vi "HFRR ADV v026 new software.vi"() -> ()   [LabVIEW 2025] (continued)
                n2409 = And(x=w2959, y=w2958) -> (x .and. y?=w2960:bool)
                n2410 = Not(x="Engage") -> (.not. x?=w2949:bool)
                n2411 = case shown="False" w2943 {
                  tunnel: [0.0 w2989] -> w2945
                  frame False {
                    (unwired) TRUE ("Visible")
                    n2412 = local read "Auto Start Test"() -> (w2970:bool)
                    n2413 = local write "Start Time"(TRUE ("Start Time")) -> ()
                    n2414 = property on="Stroke 2" class="DigNum (strict)"("Visible"=FALSE) -> ()  [unwired: 2 in, 2 out]
                    n2415 = case shown="False" w2970 {
                      frame False {
                        n2416 = property on="Heater Button" class="Bool (strict)"("DisabledEnum"=T18."Enabled" ("Disabled")) -> ()  [unwired: 2 in, 2 out]
                        n2417 = property on="Humidity" class="Bool (strict)"("DisabledEnum"=T18."Enabled" ("Disabled")) -> ()  [unwired: 2 in, 2 out]
                      }
                      frame True {
                      }
                    }
                    n2418 = case shown="False" "TestCompFlg" {
                      frame False {
                        n2419 = local read "StartFlg"() -> (w2978:bool)
                        n2420 = case shown="True" w2978 {
                          frame False {
                          }
                          frame True {
                            n2421 = stacked-sequence {
                              frame #0 {
                                n2422 = local read "EVENT LOG"() -> (w2982:string)
                                n2423 = call "Event Log.vi"("Content"="Test was interrupted", "EVENT LOG"=w2982) -> ("EVENT LOG"=w2983:string)  [unwired: 8 in, 1 out]
                                n2424 = local write "EVENT LOG"(w2983) -> ()
                                n2425 = property on="RUN" class="Bool (strict)"("Visible"=TRUE) -> ()  [unwired: 2 in, 2 out]
                                n2426 = property on="Auto Start Test" class="Bool (strict)"("Visible"=TRUE) -> ()  [unwired: 2 in, 2 out]
                              }
                              frame #1 {
                                w2985 = FALSE ("StartFlg")
                                n2427 = property on="Heater Button" class="Bool (strict)"("Val(Sgnl)"=FALSE ("Value (Signaling)")) -> ()  [unwired: 2 in, 2 out]
                                n2428 = local write "Heater Button"(w2985) -> ()
                                n2429 = local write "StartFlg"(w2985) -> ()
                                n2430 = local write "Humidity"(w2985) -> ()
                              }
                              frame #2 {
                                n2431 = local write "Due Write"("VC;0" ("Command")) -> ()
                              }
                              frame #3 {
                                n2432 = Wait (ms)(milliseconds to wait=u32 1500) -> ()  [unwired: 1 out]
                              }
                              frame #4 {
                                n2433 = local write "Due Write"("HE;0" ("Command")) -> ()
                              }
                            }
                          }
                        }
                      }
                      frame True {
                      }
                    }
                    n2434 = local write "String 14"("Test will autostart once parameters reach the set value." ("String 14")) -> ()
                  }
                  frame True {
                    (unwired) FALSE ("Visible")
                    n2435 = property on="Stroke 2" class="DigNum (strict)"("Visible"=TRUE) -> ()  [unwired: 2 in, 2 out]
                    n2436 = property on="STOP 2" class="Bool (strict)"("Disabled"=u8 2) -> ()  [unwired: 2 in, 2 out]
                    n2437 = local write "String 14"(" Running....." ("String 14")) -> ()
                    n2438 = property on="Heater Button" class="Bool (strict)"("DisabledEnum"=T18."Disabled and Grayed Out" ("Disabled")) -> ()  [unwired: 2 in, 2 out]
                    n2439 = property on="Humidity" class="Bool (strict)"("DisabledEnum"=T18."Disabled and Grayed Out" ("Disabled")) -> ()  [unwired: 2 in, 2 out]
                    n2440 = case shown="True" "Start Time" {
                      selector: "Start Time" -> [_ w3008]
                      frame False {
                      }
                      frame True {
                        n2441 = Not(x=w3008) -> (.not. x?=w3007:bool)
                        n2442 = local write "Start Time"(w3007) -> ()
                        n2443 = local read "EVENT LOG"() -> (w3009:string)
                        n2444 = call "Event Log.vi"("Content"="Test in progress", "EVENT LOG"=w3009) -> ("EVENT LOG"=w3011:string)  [unwired: 8 in, 1 out]
                        n2445 = local write "EVENT LOG"(w3011) -> ()
                      }
                    }
                    n2446 = disable-structure shown="Enabled" {
                      disable-tunnel: [w3000 w3006] -> w2989
                      frame Disabled {
                        n2447 = local read "Set Hz"() -> (w3003:dbl)
                        n2448 = call <vilib>:"Uniform White Noise Waveform.vi"() -> ("signal out"=w3002:waveform(dbl))  [unwired: 10 in, 1 out]
                        n2449 = Random Number (0-1)() -> (number: 0 to 1=w2999:dbl)
                        n2450 = Add(x=w3003, y=w3002) -> (x+y=w3001:waveform(dbl))
                        n2451 = Multiply(x=ext 0.01 ("y"), y=w2999) -> (x*y=w2997:ext)
                        n2452 = Multiply(x=w3001, y=w2997) -> (x*y=w3000:waveform(ext))
                      }
                      frame Enabled {
                        n2453 = call-poly <vilib>:"Random Number (Range).vi"("lower bound (0)"=49.89, "upper bound (100)"=50.8) -> ("number"=w3006:dbl)  [unwired: 9 in]
                      }
                    }
                    "StartFlg" <- TRUE ("StartFlg")
                  }
                }
                n2454 = case shown="True" w2960 {
                  frame False {
                  }
                  frame True {
                    n2455 = local write "clk"(10.0 ("clk")) -> ()
                    n2456 = Get Date/Time In Seconds() -> (seconds since 1Jan1904=w3014:timestamp)
                    n2457 = To Double Precision Float(number=w3014) -> (double precision float=w3012:dbl)
                    n2458 = local write "acq timer"(w3012) -> ()
                    n2459 = local write "act save time"(w3012) -> ()
                  }
                }
                n2460 = call "Elapsed Time"("Time Target (s)"="Countdown", "Reset"=w2949) -> ("Elapsed Time (s)"=w2954:dbl, "Time has Elapsed"=w2952:bool)  [unwired: 10 in, 6 out]
                "Countdown 2" <- w2954
                n2461 = Subtract(x=w2954, y=2.0) -> (x-y=w2957:dbl)
                n2462 = Less?(x=w2957, y="Countdown") -> (x < y?=w2955:bool)
                n2463 = And(x=w2955, y=w2952) -> (x .and. y?=w2951:bool)
                n2464 = case shown="True" w2951 {
                  frame False {
                  }
                  frame True {
                    (unwired) dbl[] [] ("History Data")
                    n2465 = local write "Engage"(FALSE ("Engage")) -> ()
                    n2466 = local write "RUN"(TRUE ("RUN")) -> ()
                    n2467 = local read "Humidity ( %RH )"() -> (→"Rh Before":dbl)
                  }
                }
                n2468 = local read "Test \nStatus"() -> (w2947:bool)
                n2469 = Select(t=w2945, s=w2947, f=0.0) -> (s? t:f=w2946:dbl)
                n2470 = local write "Frequency ( Hz )"(w2946) -> ()
              }
              frame #1 {
                w3037 = 1000000.0 ("x")
                # "HC;1/0\nST;VALUE"
                # "Elapsed time\ncof\nstroke\nAir temp\nTemp\nHumidity"
                # "acq timer\n\nact save time"
                # "convert to microseconds"
                n2471 = local read "COUNT"() -> (w3020:i32)
                n2472 = local read "Rate"() -> (w3033:dbl)
                n2473 = Divide(x=w3037, y=w3033) -> (x/y=w3038:dbl)
                n2474 = Greater Or Equal?(x=w3020, y=250) -> (x >= y?=w3019:bool)
                n2475 = Get Date/Time In Seconds() -> (seconds since 1Jan1904=w3040:timestamp)
                n2476 = case shown="True" w3019 {
                  frame False {
                    n2477 = local read "COUNT"() -> (w3041:i32)
                    n2478 = Increment(x=w3041) -> (x+1=w3042:i32)
                    n2479 = local write "COUNT"(w3042) -> ()
                  }
                  frame True {
                    n2480 = local write "COUNT"(0 ("COUNT")) -> ()
                  }
                }
                n2481 = local read "Samplingtime 2"() -> (w3018:dbl)
                n2482 = local read "act save time"() -> (w3035:dbl)
                n2483 = Divide(x=w3038, y=w3037) -> (x/y=w3036:dbl)
                n2484 = To Double Precision Float(number=w3040) -> (double precision float=w3029:dbl)
                n2485 = Add(x=w3035, y=w3018) -> (x+y=w3034:dbl)
                n2486 = local read "acq timer"() -> (w3039:dbl)
                n2487 = local read "COUNT"() -> (w3022:i32)
                n2488 = Greater Or Equal?(x=w3029, y=w3034) -> (x >= y?=w3017:bool)
                n2489 = Multiply(x=w3036, y=w3022) -> (x*y=w3028:dbl)
                n2490 = Subtract(x=w3029, y=w3039) -> (x-y=w3031:dbl)
                n2491 = local read "Save"() -> (w3032:bool)
                n2492 = Add(x=w3031, y=w3028) -> (x+y=w3015:dbl)
                "Elapsed time 3" <- w3015
                n2493 = And(x=w3017, y=w3032) -> (x .and. y?=w3030:bool)
                n2494 = Divide(x=w3015, y=60.0) -> (x/y=w3026:dbl)
                n2495 = local read "Test \nStatus"() -> (w3016:bool)
                n2496 = local read "clk"() -> (w3023:dbl)
                n2497 = Equal?(x=w3023, y=10.0) -> (x = y?=w3025:bool)
                n2498 = case shown="True" w3030 {
                  tunnel: w3029 -> [_ w3153]
                  tunnel: [FALSE ("Boolean 2") TRUE ("Boolean 2")] -> _
                  frame False {
                  }
                  frame True {
                    w3107 = ";" ("Substring")
                    # "Pid out/\nFreq response value"
                    n2499 = local write "act save time"(w3153) -> ()
                    n2500 = local read "FILE"() -> (w3101:string)
                    n2501 = call "file check.vi"("file name in"=w3101) -> ("error out"=w3104:errorcluster, "file name out"=w3099:string)  [unwired: 9 in]
                    n2502 = local read "LVDT STROKE"() -> (w3096:dbl)
                    n2503 = local read "Add up Stroke"() -> (w3094:dbl)
                    n2504 = call "FILE PATH CREATION.vi"("error in"=w3104, "FILE NAME :"=w3099) -> ("FILE OUT"=w3102:path)  [unwired: 8 in, 1 out]
                    n2505 = Concatenate Strings(w3099, ".dgf" ("Substring")) -> (w3103:string)
                    n2506 = Subtract(x=w3096, y=w3094) -> (x-y=w3095:dbl)
                    n2507 = Absolute Value(x=w3095) -> (abs(x)=w3093:dbl)
                    n2508 = local read "FF 2"() -> (→"Frictional Force ( N )" →"Frictional Force ( N )":dbl)
                    n2509 = Build Path(base path=w3102, name or relative path=w3103) -> (appended path=w3098:path)
                    n2510 = local read "COF 2"() -> (w3112:dbl)
                    "Coefficient of Friction" <- w3112
                    "COF 4" <- w3112
                    "Coefficient of Friction" <- w3112
                    n2511 = local read "TEMP"() -> (w3115:dbl)
                    "Temperature ( Deg C )" <- w3115
                    n2512 = local read "Humidity ( %RH )"() -> (w3114:dbl)
                    "Humidity ( %RH )" <- w3114
                    "Humidity ( %RH )" <- w3114
                    n2513 = local read "Frequency ( Hz )"() -> (w3121:dbl)
                    n2514 = call <vilib>:"Mean PtByPt.vi"("x"=w3093, "sample length"="STROKE FILTER") -> ("mean"=w3092:dbl)  [unwired: 2 in, 1 out]
                    n2515 = local read "Elapsed time"() -> (w3146:dbl)
                    n2516 = local read "AIR TEMP"() -> (w3119:dbl)
                    n2517 = local read "PID-out"() -> (w3124:dbl)
                    n2518 = local write "Temperature ( Deg C )"(w3115) -> ()
                    n2519 = Number To Fractional String(number=w3092, width (-)=i16 9 ("precision (6)"), precision (6)=i16 6) -> (F-format string=w3139:string)  [unwired: 1 in]
                    n2520 = Number To Fractional String(number=w3119, width (-)=i16 9 ("precision (6)"), precision (6)=i16 3) -> (F-format string=w3138:string)  [unwired: 1 in]
                    n2521 = Number To Fractional String(number=w3115, width (-)=i16 9 ("precision (6)"), precision (6)=i16 3) -> (F-format string=w3135:string)  [unwired: 1 in]
                    n2522 = Number To Fractional String(number=w3114, width (-)=i16 9 ("precision (6)"), precision (6)=i16 3) -> (F-format string=w3132:string)  [unwired: 1 in]
                    n2523 = Number To Fractional String(number=0.0, width (-)=i16 9 ("precision (6)"), precision (6)=i16 3) -> (F-format string=w3129:string)  [unwired: 1 in]
                    n2524 = Number To Fractional String(number=w3124, width (-)=i16 9 ("precision (6)"), precision (6)=i16 3) -> (F-format string=w3125:string)  [unwired: 1 in]
                    n2525 = Number To Fractional String(number=w3121, width (-)=i16 9 ("precision (6)"), precision (6)=i16 3) -> (F-format string=w3120:string)  [unwired: 1 in]
                    n2526 = Number To Fractional String(number=w3112, width (-)=i16 9 ("precision (6)"), precision (6)=i16 6) -> (F-format string=w3147:string)  [unwired: 1 in]
                    n2527 = Number To Fractional String(number=w3146, width (-)=i16 14 ("precision (6)"), precision (6)=i16 3) -> (F-format string=w3148:string)  [unwired: 1 in]
                    n2528 = Bundle("y"=1.02, "mean"=w3092, "y"=0.98) -> (w3113:cluster{"y":dbl, "mean":dbl, "y":dbl})  [unwired: 1 in]
                    n2529 = Number To Fractional String(number="Ambient Humidity :", width (-)=i16 9 ("precision (6)"), precision (6)=i16 6) -> (F-format string=w3105:string)  [unwired: 1 in]
                    n2530 = local read "RUN"() -> (w3111:bool)
                    n2531 = case shown="True" w3111 {
                      tunnel: w3113 -> [_ w3158]
                      tunnel: w3092 -> [_ w3157]
                      tunnel: w3092 -> [_ w3155]
                      tunnel: w3092 -> [_ w3156]
                      frame False {
                      }
                      frame True {
                        "Stroke ( mm )" <- w3158
                        "Stroke ( mm )" <- w3158
                        "Stroke 4" <- w3157
                        "Stroke 3" <- w3155
                        "Stroke 2" <- w3156
                        "measured_stroke" <- w3155
                      }
                    }
                    n2532 = Concatenate Strings(w3148, w3107, w3147, w3107, w3139, w3107, w3138, w3107, w3135, w3107, w3132, w3107, w3129, w3107, w3125, w3107, w3120, w3107, w3105, "\r") -> (w3145:string)
                    n2533 = call <vilib>:"Write Characters To File.vi"("append to file? (new file:F)"=TRUE, "character string"=w3145, "file path (dialog if empty)"=w3098) -> ()  [unwired: 2 in, 1 out]
                    "refresh flag" <- TRUE ("refresh flag")
                  }
                }
                n2534 = case shown="True" w3016 {
                  tunnel: w3026 -> [_ w3052]
                  tunnel: w3031 -> [_ w3062]
                  tunnel: [0.0 w3058] -> _
                  tunnel: w3025 -> [_ w3057]
                  tunnel: [0.0 w3056] -> _
                  tunnel: w3015 -> [_ w3056]
                  tunnel: w3029 -> [w3045 _]
                  frame False {
                    n2535 = local write "acq timer"(w3045) -> ()
                    n2536 = local write "Test Duration Status"(0.0 ("Test Duration Status")) -> ()
                  }
                  frame True {
                    n2537 = local read "Set Hz"() -> (w3059:dbl)
                    n2538 = local write "Elapsed time"(w3052) -> ()
                    n2539 = local read "test time"() -> (w3051:dbl)
                    n2540 = Multiply(x=w3062, y=w3059) -> (x*y=w3061:dbl)
                    n2541 = case shown="False" w3057 {
                      tunnel: w3061 -> [w3063 _]
                      tunnel: [w3063 1.0] -> w3058
                      frame False {
                        n2542 = local write "Cycles elapsed"(w3063) -> ()
                      }
                      frame True {
                      }
                    }
                    n2543 = Greater?(x=w3052, y=w3051) -> (0:w3060:bool)
                    n2544 = Subtract(x=w3051, y=w3052) -> (x-y=w3050:dbl)
                    n2545 = Multiply(x=w3050, y=60.0) -> (x*y=w3049:dbl)
                    n2546 = local write "Time Remaining"(w3049) -> ()
                    n2547 = local write "Remaining Time"(w3049) -> ()
                    n2548 = case shown="True" w3060 {
                      frame False {
                      }
                      frame True {
                        n2549 = stacked-sequence {
                          frame #0 {
                            w3068 = T18."Enabled" ("Disabled")
                            w3067 = FALSE ("TEST FILE NAM,E SAVED")
                            w3069 = "" ("FILE")
                            w3070 = TRUE ("Visible")
                            n2550 = local write "Humidity"(FALSE ("Humidity")) -> ()
                            n2551 = local write "RUN"(FALSE ("OK Button 2")) -> ()
                            n2552 = local write "Heater Button"(FALSE ("Heater Button")) -> ()
                            n2553 = local write "Auto Start Test"(FALSE ("Auto Start Test")) -> ()
                            n2554 = local write "TestCompFlg"(TRUE ("StpFlg")) -> ()
                            n2555 = local read "Humidity ( %RH )"() -> (→"Rh After":dbl)
                            n2556 = property on="STOP 2" class="Bool (strict)"("Disabled"=u8 0) -> ()  [unwired: 2 in, 2 out]
                            n2557 = local read "EVENT LOG"() -> (w3075:string)
                            n2558 = call "Event Log.vi"("Content"="Test Completed", "EVENT LOG"=w3075) -> ("EVENT LOG"=w3074:string)  [unwired: 8 in, 1 out]
                            n2559 = property on="RUN" class="Bool (strict)"("Visible"=w3070) -> ()  [unwired: 2 in, 2 out]
                            n2560 = property on="Auto Start Test" class="Bool (strict)"("Visible"=w3070) -> ()  [unwired: 2 in, 2 out]
                            n2561 = local write "Batch Ref Num :"(w3069) -> ()
                            n2562 = local write "FILE"(w3069) -> ()
                            n2563 = local write "EVENT LOG"(w3074) -> ()
                            n2564 = local write "TEST FILE NAM,E SAVED"(w3067) -> ()
                            n2565 = local write "Fuel Discription :"(w3069) -> ()
                            n2566 = local write "START TEMP"(w3067) -> ()
                            n2567 = local write "Remarks :"(w3069) -> ()
                            n2568 = local write "Main Dashboard Buttons"(T1."Imaging" ("Main Dashboard Buttons")) -> ()
                            n2569 = local write "Main Tab"(T2."Adv Scar" ("Main Tab")) -> ()
                            n2570 = property on="FRICVALZ 2" class="Bool (strict)"("DisabledEnum"=w3068) -> ()  [unwired: 2 in, 2 out]
                            n2571 = property on="FRICVALZ 3" class="Bool (strict)"("DisabledEnum"=w3068) -> ()  [unwired: 2 in, 2 out]
                            n2572 = property on="FRICVALZ 4" class="Bool (strict)"("DisabledEnum"=w3068) -> ()  [unwired: 2 in, 2 out]
                          }
                          frame #1 {
                            n2573 = Wait (ms)(milliseconds to wait=u32 1500) -> ()  [unwired: 1 out]
                          }
                          frame #2 {
                            n2574 = local write "Due Write"("VC;0") -> ()
                          }
                          frame #3 {
                            n2575 = Wait (ms)(milliseconds to wait=u32 1500) -> ()  [unwired: 1 out]
                          }
                          frame #4 {
                            n2576 = local write "Due Write"("VC;0") -> ()
                          }
                          frame #5 {
                            n2577 = Wait (ms)(milliseconds to wait=u32 1500) -> ()  [unwired: 1 out]
                          }
                          frame #6 {
                            n2578 = local write "Due Write"("ST;0") -> ()
                          }
                          frame #7 {
                            n2579 = local write "measured_stroke"(0.0 ("measured_stroke")) -> ()
                            n2580 = Wait (ms)(milliseconds to wait=u32 1500) -> ()  [unwired: 1 out]
                          }
                          frame #8 {
                            n2581 = local write "Due Write"("HE;0") -> ()
                          }
                        }
                      }
                    }
                    n2582 = Divide(x=w3052, y=w3051) -> (x/y=w3055:dbl)
                    n2583 = Multiply(x=w3055, y=100.0) -> (x*y=w3053:dbl)
                    n2584 = local write "Test Duration Status"(w3053) -> ()
                  }
                }
              }
              frame #2 {
                n2585 = case shown="True" "Heater Button" {
                  tunnel: [0.0 ("output") w3181] -> w3159
                  frame False {
                    w3162 = TRUE ("tmpchk")
                    n2586 = local read "TEMP"() -> (w3163:dbl)
                    n2587 = local write "Temp ini"(w3163) -> ()
                    n2588 = local write "Reset 4"(w3162) -> ()
                    n2589 = local write "tmpchk"(w3162) -> ()
                    n2590 = local write "reinit"(TRUE ("reinit")) -> ()
                    n2591 = local write "manual temp log"(TRUE ("manual temp log")) -> ()
                  }
                  frame True {
                    # "Logic to turn off\nthe heater when \ntemp is not rising.\nTime - 60 sec\nDelta t- 5°c"
                    n2592 = local read "Temp ini"() -> (w3170:dbl)
                    n2593 = local read "Auto Start Test"() -> (w3166:bool)
                    n2594 = Less?(x=w3170, y=53.0) -> (x < y?=w3168:bool)
                    n2595 = case shown="False" w3166 {
                      frame False {
                        n2596 = local read "Set Temp"() -> (w3190:dbl)
                        n2597 = local read "TEMP"() -> (w3189:dbl)
                        n2598 = Subtract(x=w3190, y=w3189) -> (x-y=w3188:dbl)
                        n2599 = Absolute Value(x=w3188) -> (abs(x)=w3187:dbl)
                        n2600 = Less?(x=w3187, y=0.5) -> (x < y?=w3185:bool)
                        n2601 = case shown="True" w3185 {
                          tunnel: "manual temp log" -> [_ w3191]
                          frame False {
                          }
                          frame True {
                            n2602 = case shown="True" w3191 {
                              selector: w3191 -> [_ w3192]
                              frame False {
                              }
                              frame True {
                                # "#Event log"
                                n2603 = Not(x=w3192) -> (.not. x?=w3193:bool)
                                n2604 = local write "manual temp log"(w3193) -> ()
                                n2605 = local read "EVENT LOG"() -> (w3196:string)
                                n2606 = call "Event Log.vi"("Content"="Target Temperature reached", "EVENT LOG"=w3196) -> ("EVENT LOG"=w3195:string)  [unwired: 8 in, 1 out]
                                n2607 = local write "EVENT LOG"(w3195) -> ()
                              }
                            }
                          }
                        }
                      }
                      frame True {
                        n2608 = local write "manual temp log"(TRUE ("manual temp log")) -> ()
                      }
                    }
                    n2609 = And(x="tmpchk", y=w3168) -> (x .and. y?=w3171:bool)
                    n2610 = case shown="True" w3171 {
                      frame False {
                      }
                      frame True {
                        n2611 = call "Elapsed Time8"("Time Target (s)"=300.0, "Reset"="Reset 4") -> ("Time has Elapsed"=w3198:bool)  [unwired: 10 in, 7 out]
                        n2612 = flat-sequence {
                          tunnel: w3198 -> [_]
                          frame #0 {
                            n2613 = local write "Reset 4"(FALSE ("Reset 4")) -> ()
                          }
                        }
                        n2614 = case shown="True" w3198 {
                          frame False {
                          }
                          frame True {
                            n2615 = local read "Temp ini"() -> (w3205:dbl)
                            n2616 = Add(x=w3205, y=5.0) -> (x+y=w3203:dbl)
                            n2617 = local read "TEMP"() -> (w3206:dbl)
                            n2618 = Greater?(x=w3206, y=w3203) -> (0:w3204:bool)
                            n2619 = case shown="False" w3204 {
                              frame False {
                                n2620 = local write "Heater Button"(FALSE ("Heater Button")) -> ()
                              }
                              frame True {
                                n2621 = local write "tmpchk"(FALSE ("tmpchk")) -> ()
                              }
                            }
                          }
                        }
                      }
                    }
                    n2622 = local read "Set Temp"() -> (w3179:dbl)
                    n2623 = local read "TEMP"() -> (w3173:dbl)
                    n2624 = call-poly <vilib>:"PID.vi"("reinitialize? (F)"="reinit", "dt (s)"=-1.0, "process variable"=w3173, "setpoint"=w3179) -> ("output"=w3176:dbl)  [unwired: 6 in, 1 out]
                    n2625 = Subtract(x=w3179, y=w3173) -> (x-y=w3180:dbl)
                    n2626 = Add(x=w3179, y=0.5) -> (x+y=w3177:dbl)
                    n2627 = Greater Or Equal?(x=w3173, y=w3177) -> ()  [unwired: 1 out]
                    n2628 = Select(t=0.0, s=FALSE, f=w3176) -> (s? t:f=w3175:dbl)
                    "PID output" <- w3175
                    n2629 = flat-sequence {
                      tunnel: w3175 -> [w3209]
                      tunnel: [w3209] -> w3181
                      frame #0 {
                        n2630 = local write "reinit"(FALSE ("reinit")) -> ()
                      }
                    }
                    n2631 = Bundle(w3180, "output"=w3175, "TEMP"=w3173) -> ()  [unwired: 1 in, 1 out]
                  }
                }
                "PID-out" <- w3159
              }
              frame #3 {
                n2632 = local read "TEMP"() -> (w3211:dbl)
                n2633 = Greater Or Equal?(x=w3211, y="Set Temp 2") -> (x >= y?=w3216:bool)
                n2634 = case shown="True" w3216 {
                  tunnel: [FALSE TRUE] -> w3214
                  frame False {
                  }
                  frame True {
                  }
                }
                "Status 13" <- w3214
                n2635 = And(x=w3214, y="trip1 8") -> (x .and. y?=w3213:bool)
                n2636 = case shown="True" w3213 {
                  frame False {
                    n2637 = local write "Heater Trip Temp"(TRUE ("Heater Trip Temp")) -> ()
                  }
                  frame True {
                    w3219 = FALSE ("OK Button 2")
                    n2638 = case shown="True" "Heater Trip Temp" {
                      selector: "Heater Trip Temp" -> [_ w3221]
                      frame False {
                      }
                      frame True {
                        n2639 = Not(x=w3221) -> (.not. x?=w3220:bool)
                        n2640 = local read "EVENT LOG"() -> (w3224:string)
                        n2641 = local write "Heater Trip Temp"(w3220) -> ()
                        n2642 = call "Event Log.vi"("Content"="Heater Trip", "EVENT LOG"=w3224) -> ("EVENT LOG"=w3223:string)  [unwired: 8 in, 1 out]
                        n2643 = local write "EVENT LOG"(w3223) -> ()
                      }
                    }
                    n2644 = local write "RUN"(w3219) -> ()
                    n2645 = property on="Auto Start Test" class="Bool (strict)"("Value"=w3219) -> ()  [unwired: 2 in, 2 out]
                    n2646 = local write "Heater Button"(w3219) -> ()
                  }
                }
              }
            }
            n2647 = case shown="False" w2940 {
              frame False {
                n2648 = disable-structure shown="Disabled" {
                  frame Disabled {
                    n2649 = stacked-sequence {
                      frame #0 {
                        n2650 = local write "RUN"(FALSE ("OK Button 2")) -> ()
                      }
                      frame #1 {
                      }
                    }
                  }
                  frame Enabled {
                  }
                }
              }
              frame True {
              }
            }
          }
        }
        n2651 = local read "Reset Graph"() -> (w2830:bool)
        n2652 = case shown="True" w2830 {
          selector: w2830 -> [_ w2847]
          frame False {
          }
          frame True {
            w2861 = 0.0 ("X Scale.Range:Maximum")
            n2653 = Not(x=w2847) -> (.not. x?=w2846:bool)
            n2654 = local write "Reset Graph"(w2846) -> ()
            n2655 = property on="Electrical Contact Resistance ( % )" class="WFChart (strict)"("XScale.Maximum"=600.0 ("X Scale.Range:Maximum"), "XScale.Minimum"=0.0 ("X Scale.Range:Minimum"), "YScale.Maximum"=100.0 ("Y Scale.Range:Maximum"), "YScale.Minimum"=0.0 ("Y Scale.Range:Minimum")) -> ()  [unwired: 2 in, 2 out]
            n2656 = property on="Frictional Force ( N )" class="WFChart (strict)"("XScale.Maximum"=600.0 ("X Scale.Range:Maximum"), "XScale.Minimum"=0.0 ("X Scale.Range:Minimum"), "YScale.Maximum"=100.0 ("Y Scale.Range:Maximum"), "YScale.Minimum"=0.0 ("Y Scale.Range:Minimum")) -> ()  [unwired: 2 in, 2 out]
            n2657 = property on="Temperature ( Deg C )" class="WFChart (strict)"("XScale.Maximum"=600.0 ("X Scale.Range:Maximum"), "XScale.Minimum"=0.0 ("X Scale.Range:Minimum"), "YScale.Maximum"=100.0 ("Y Scale.Range:Maximum"), "YScale.Minimum"=0.0 ("Y Scale.Range:Minimum")) -> ()  [unwired: 2 in, 2 out]
            n2658 = property on="Humidity ( %RH )" class="WFChart (strict)"("XScale.Maximum"=600.0 ("X Scale.Range:Maximum"), "XScale.Minimum"=0.0 ("X Scale.Range:Minimum"), "YScale.Maximum"=100.0 ("Y Scale.Range:Maximum"), "YScale.Minimum"=0.0 ("Y Scale.Range:Minimum")) -> ()  [unwired: 2 in, 2 out]
            n2659 = property on="Stroke ( mm )" class="WFChart (strict)"("XScale.Maximum"=600.0 ("X Scale.Range:Maximum"), "XScale.Minimum"=0.0 ("X Scale.Range:Minimum"), "YScale.Maximum"=100.0 ("Y Scale.Range:Maximum"), "YScale.Minimum"=0.0 ("Y Scale.Range:Minimum")) -> ()  [unwired: 2 in, 2 out]
            n2660 = property on="Coefficient of Friction" class="WFChart (strict)"("XScale.Maximum"=600.0 ("X Scale.Range:Maximum"), "XScale.Minimum"=0.0 ("X Scale.Range:Minimum"), "YScale.Maximum"=100.0 ("Y Scale.Range:Maximum"), "YScale.Minimum"=0.0 ("Y Scale.Range:Minimum")) -> ()  [unwired: 2 in, 2 out]
            n2661 = property on="Electrical Contact Resistance ( % )" class="WFChart (strict)"("XScale.Minimum"=0.0 ("X Scale.Range:Minimum"), "XScale.Maximum"=600.0 ("X Scale.Range:Maximum"), "YScale.Minimum"=0.0 ("Y Scale.Range:Minimum"), "YScale.Maximum"=100.0 ("Y Scale.Range:Maximum")) -> ()  [unwired: 2 in, 2 out]
            n2662 = property on="Temperature ( Deg C )" class="WFChart (strict)"("XScale.Minimum"=0.0 ("X Scale.Range:Minimum"), "XScale.Maximum"=600.0 ("X Scale.Range:Maximum"), "YScale.Minimum"=0.0 ("Y Scale.Range:Minimum"), "YScale.Maximum"=100.0 ("Y Scale.Range:Maximum")) -> ()  [unwired: 2 in, 2 out]
            n2663 = property on="Coefficient of Friction" class="WFChart (strict)"("XScale.Minimum"=0.0 ("X Scale.Range:Minimum"), "XScale.Maximum"=600.0 ("X Scale.Range:Maximum"), "YScale.Maximum"=1.0 ("X Scale.Range:Minimum"), "YScale.Minimum"=0.0 ("X Scale.Range:Minimum")) -> ()  [unwired: 2 in, 2 out]
            n2664 = property on="Frictional Force ( N )" class="WFChart (strict)"("XScale.Maximum"=600.0 ("X Scale.Range:Maximum"), "XScale.Minimum"=w2861, "YScale.Maximum"=10.0 ("Y Scale.Range:Maximum"), "YScale.Minimum"=w2861) -> ()  [unwired: 2 in, 2 out]
            n2665 = property on="Stroke ( mm )" class="WFChart (strict)"("XScale.Maximum"=600.0 ("X Scale.Range:Maximum"), "XScale.Minimum"=0.0 ("X Scale.Range:Minimum"), "YScale.Maximum"=100.0 ("Y Scale.Range:Maximum"), "YScale.Minimum"=0.0 ("Y Scale.Range:Minimum")) -> ()  [unwired: 2 in, 2 out]
            n2666 = property on="Humidity ( %RH )" class="WFChart (strict)"("XScale.Maximum"=600.0 ("X Scale.Range:Maximum"), "XScale.Minimum"=0.0 ("X Scale.Range:Minimum"), "YScale.Maximum"=100.0 ("Y Scale.Range:Maximum"), "YScale.Minimum"=0.0 ("Y Scale.Range:Minimum")) -> ()  [unwired: 2 in, 2 out]
          }
        }
      }
      frame "Compare Files" {
        # "Elapsed time\ncof\nstroke\nAir temp\nTemp\nHumidity"
        n2667 = case shown="True" "RSTV1 2" {
          frame False {
          }
          frame True {
            n2668 = property on="Humidity ( %RH )" class="XYGraph (strict)"("Y Scale.Display Format:Precision"=u8 0 ("Y Scale.Format & Precision:Precision")) -> ()  [unwired: 2 in, 2 out]
            n2669 = property on="Humidity ( %RH )" class="XYGraph (strict)"("X Scale.Range:Minimum"=0.0, "X Scale.Range:Maximum"=75.0, "Y Scale.Range:Minimum"=48.0, "Y Scale.Range:Maximum"=58.0) -> ()  [unwired: 2 in, 2 out]
          }
        }
        n2670 = case shown="True" "RST CP 2" {
          frame False {
          }
          frame True {
            n2671 = property on="XY Graph 13" class="XYGraph (strict)"("Y Scale.Display Format:Precision"=u8 0 ("Y Scale.Format & Precision:Precision")) -> ()  [unwired: 2 in, 2 out]
            n2672 = property on="XY Graph 13" class="XYGraph (strict)"("X Scale.Range:Minimum"=0.0, "X Scale.Range:Maximum"=75.0, "Y Scale.Range:Minimum"=0.0, "Y Scale.Range:Maximum"=100.0) -> ()  [unwired: 2 in, 2 out]
          }
        }
        n2673 = case shown="True" "RST CP" {
          frame False {
          }
          frame True {
            n2674 = property on="Sample Temperature ( °C )" class="XYGraph (strict)"("Y Scale.Display Format:Precision"=u8 2 ("Y Scale.Format & Precision:Precision")) -> ()  [unwired: 2 in, 2 out]
            n2675 = property on="Sample Temperature ( °C )" class="XYGraph (strict)"("X Scale.Range:Minimum"=0.0, "X Scale.Range:Maximum"=75.0, "Y Scale.Range:Minimum"=58.0, "Y Scale.Range:Maximum"=62.0) -> ()  [unwired: 2 in, 2 out]
          }
        }
        n2676 = case shown="True" "RSTV1 3" {
          frame False {
          }
          frame True {
            n2677 = property on="Air Temperature  ( °C )" class="XYGraph (strict)"("Y Scale.Display Format:Precision"=u8 2 ("Y Scale.Format & Precision:Precision")) -> ()  [unwired: 2 in, 2 out]
            n2678 = property on="Air Temperature  ( °C )" class="XYGraph (strict)"("X Scale.Range:Minimum"=0.0 ("Y Scale.Range:Minimum"), "X Scale.Range:Maximum"=75.0 ("Y Scale.Range:Maximum"), "Y Scale.Range:Minimum"=20.0 ("X Scale.Range:Minimum"), "Y Scale.Range:Maximum"=26.0 ("X Scale.Range:Maximum")) -> ()  [unwired: 2 in, 2 out]
          }
        }
        n2679 = case shown="True" "RSTV1 4" {
          frame False {
          }
          frame True {
            n2680 = property on="Stroke ( mm )" class="XYGraph (strict)"("Y Scale.Display Format:Precision"=u8 2 ("Y Scale.Format & Precision:Precision")) -> ()  [unwired: 2 in, 2 out]
            n2681 = property on="Stroke ( mm )" class="XYGraph (strict)"("X Scale.Range:Minimum"=0.0 ("Y Scale.Range:Maximum"), "X Scale.Range:Maximum"=75.0 ("X Scale.Range:Minimum"), "Y Scale.Range:Minimum"=0.98, "Y Scale.Range:Maximum"=1.02) -> ()  [unwired: 2 in, 2 out]
          }
        }
        n2682 = case shown="True" "rstv2" {
          frame False {
          }
          frame True {
            n2683 = property on="Coefficient Of Friction" class="XYGraph (strict)"("Y Scale.Display Format:Precision"=u8 3 ("Y Scale.Format & Precision:Precision")) -> ()  [unwired: 2 in, 2 out]
            n2684 = property on="Coefficient Of Friction" class="XYGraph (strict)"("X Scale.Range:Minimum"=0.0 ("Y Scale.Range:Maximum"), "X Scale.Range:Maximum"=75.0, "Y Scale.Range:Minimum"=0.0, "Y Scale.Range:Maximum"=1.0 ("X Scale.Range:Minimum")) -> ()  [unwired: 2 in, 2 out]
          }
        }
        n2685 = case shown="True" "RST CP 3" {
          frame False {
          }
          frame True {
            n2686 = property on="Air Temp ( °C ) vs Humidity ( % RH )" class="XYGraph (strict)"("X Scale.Range:Minimum"=18.0, "X Scale.Range:Maximum"=28.0 ("X Scale.Range:Minimum"), "Y Scale.Range:Minimum"=30.0 ("X Scale.Range:Minimum"), "Y Scale.Range:Maximum"=70.0 ("X Scale.Range:Minimum")) -> ()  [unwired: 2 in, 2 out]
          }
        }
        n2687 = case shown="True" "OPEN 1" {
          frame False {
          }
          frame True {
            (unwired) 0  # existing file
            w3500 = "Choose a datalog file to open"  # prompt
            n2688 = local write "OPEN 1"(FALSE ("OPEN 1")) -> ()
            n2689 = String To Path(string="C:\\LAB-IQ\\Data\\") -> (path=w3485:path)
            n2690 = File Dialog(6:"*.dgf" ("pattern"), 7:w3500, 11:w3485) -> (0:w3483:errorcluster, 3:w3491:path)  [unwired: 4 in, 2 out]
            n2691 = Unbundle(w3483) -> ()  [unwired: 3 out]
            n2692 = Strip Path(path=w3491) -> (name=w3490:string)  [unwired: 1 out]
            n2693 = Path To String(path=w3491) -> (string=w3486:string)
            "string1" <- w3486
            n2694 = Match Pattern(string=w3490, regular expression=".dgf") -> (before substring=→"String Control":string)  [unwired: 1 in, 3 out]
            n2695 = Match Pattern(string=w3486, regular expression=".dgf" ("substring (\"\")")) -> (before substring=w3496:string)  [unwired: 1 in, 3 out]
            n2696 = Concatenate Strings(w3496, ".duf" ("Substring")) -> (w3492:string)
            n2697 = String To Path(string=w3492) -> (path=w3497:path)
            n2698 = call <vilib>:"Read Characters From File.vi"("file path (dialog if empty)"=w3497, "start of read offset (chars.:0)"=60 ("start of read offset (chars.: 0)")) -> ("character string"=→"String Control 2":string)  [unwired: 4 in, 3 out]
          }
        }
        n2699 = case shown="True" "OPEN 2" {
          frame False {
          }
          frame True {
            (unwired) 0  # existing file
            w3518 = "Choose a datalog file to open"  # prompt
            n2700 = local write "OPEN 2"(FALSE ("OPEN 1")) -> ()
            n2701 = String To Path(string="C:\\LAB-IQ\\Data\\") -> (path=w3503:path)
            n2702 = File Dialog(6:"*.dgf" ("pattern"), 7:w3518, 11:w3503) -> (0:w3501:errorcluster, 3:w3509:path)  [unwired: 4 in, 2 out]
            n2703 = Unbundle(w3501) -> ()  [unwired: 3 out]
            n2704 = Strip Path(path=w3509) -> (name=w3507:string)  [unwired: 1 out]
            n2705 = Path To String(path=w3509) -> (string=w3504:string)
            "string1 2" <- w3504
            n2706 = Match Pattern(string=w3507, regular expression=".dgf") -> (before substring=→"String Control 3":string)  [unwired: 1 in, 3 out]
            n2707 = Match Pattern(string=w3504, regular expression=".dgf" ("substring (\"\")")) -> (before substring=w3515:string)  [unwired: 1 in, 3 out]
            n2708 = Concatenate Strings(w3515, ".duf" ("Substring")) -> (w3512:string)
            n2709 = String To Path(string=w3512) -> (path=w3510:path)
            n2710 = call <vilib>:"Read Characters From File.vi"("file path (dialog if empty)"=w3510, "start of read offset (chars.:0)"=60 ("start of read offset (chars.: 0)")) -> ("character string"=→"String Control 4":string)  [unwired: 4 in, 3 out]
          }
        }
        n2711 = case shown="True" "OPEN 3" {
          frame False {
          }
          frame True {
            (unwired) 0  # existing file
            w3536 = "Choose a datalog file to open"  # prompt
            n2712 = local write "OPEN 3"(FALSE ("OPEN 1")) -> ()
            n2713 = String To Path(string="C:\\LAB-IQ\\Data\\") -> (path=w3521:path)
            n2714 = File Dialog(6:"*.dgf" ("pattern"), 7:w3536, 11:w3521) -> (0:w3519:errorcluster, 3:w3527:path)  [unwired: 4 in, 2 out]
            n2715 = Unbundle(w3519) -> ()  [unwired: 3 out]
            n2716 = Strip Path(path=w3527) -> (name=w3525:string)  [unwired: 1 out]
            n2717 = Path To String(path=w3527) -> (string=w3522:string)
            "string1 3" <- w3522
            n2718 = Match Pattern(string=w3525, regular expression=".dgf") -> (before substring=→"String Control 5":string)  [unwired: 1 in, 3 out]
            n2719 = Match Pattern(string=w3522, regular expression=".dgf" ("substring (\"\")")) -> (before substring=w3532:string)  [unwired: 1 in, 3 out]
            n2720 = Concatenate Strings(w3532, ".duf" ("Substring")) -> (w3529:string)
            n2721 = String To Path(string=w3529) -> (path=w3533:path)
            n2722 = call <vilib>:"Read Characters From File.vi"("file path (dialog if empty)"=w3533, "start of read offset (chars.:0)"=60 ("start of read offset (chars.: 0)")) -> ("character string"=→"String Control 6":string)  [unwired: 4 in, 3 out]
          }
        }
        n2723 = case shown="True" "OPEN 4" {
          frame False {
          }
          frame True {
            (unwired) 0  # existing file
            w3554 = "Choose a datalog file to open"  # prompt
            n2724 = local write "OPEN 4"(FALSE ("OPEN 1")) -> ()
            n2725 = String To Path(string="C:\\LAB-IQ\\Data\\") -> (path=w3539:path)
            n2726 = File Dialog(6:"*.dgf" ("pattern"), 7:w3554, 11:w3539) -> (0:w3537:errorcluster, 3:w3545:path)  [unwired: 4 in, 2 out]
            n2727 = Unbundle(w3537) -> ()  [unwired: 3 out]
            n2728 = Strip Path(path=w3545) -> (name=w3543:string)  [unwired: 1 out]
            n2729 = Path To String(path=w3545) -> (string=w3540:string)
            "string1 4" <- w3540
            n2730 = Match Pattern(string=w3543, regular expression=".dgf") -> (before substring=→"String Control 7":string)  [unwired: 1 in, 3 out]
            n2731 = Match Pattern(string=w3540, regular expression=".dgf" ("substring (\"\")")) -> (before substring=w3550:string)  [unwired: 1 in, 3 out]
            n2732 = Concatenate Strings(w3550, ".duf" ("Substring")) -> (w3547:string)
            n2733 = String To Path(string=w3547) -> (path=w3551:path)
            n2734 = call <vilib>:"Read Characters From File.vi"("file path (dialog if empty)"=w3551, "start of read offset (chars.:0)"=60 ("start of read offset (chars.: 0)")) -> ("character string"=→"String Control 8":string)  [unwired: 4 in, 3 out]
          }
        }
      }
      frame "About" {
        # "Elapsed time\ncof\nstroke\nmean pos\nTemp\nHumidity"
        n2735 = disable-structure shown="Disabled" {
          frame Disabled {
            n2736 = case shown="True" "Export" {
              frame False {
              }
              frame True {
                w3576 = "                                      " ("string")
                w3578 = "\r"
                (unwired) i16 6 ("width (-)")
                w3655 = "\r"
                w3587 = "\r"
                n2737 = local write "Export"(FALSE ("Export")) -> ()
                n2738 = local read "String 29"() -> (w3624:string)
                n2739 = local read "String 34"() -> (w3612:string)
                n2740 = local read "String 35"() -> (w3607:string)
                n2741 = local read "String 37"() -> (w3603:string)
                n2742 = local read "String 36"() -> (w3600:string)
                n2743 = local read "String 38"() -> (w3597:string)
                n2744 = local read "String 39"() -> (w3594:string)
                n2745 = Match Pattern(string=w3624, regular expression=".dwm") -> (before substring=w3620:string)  [unwired: 1 in, 3 out]
                "before substring" <- w3620
                n2746 = local read "S 38"() -> (w3615:string)
                n2747 = local read "S 39"() -> (w3608:string)
                n2748 = local read "Temperature before test 2"() -> (w3644:dbl)
                n2749 = local read "Temperature after test 2"() -> (w3649:dbl)
                n2750 = local read "Humidity before test 2"() -> (w3630:dbl)
                n2751 = local read "Humidity after test 2"() -> (w3645:dbl)
                n2752 = local read "MWSD 2"() -> (w3641:dbl)
                n2753 = local read "WS1.4 2"() -> (w3657:dbl)
                n2754 = local read "HCF 2"() -> (w3653:dbl)
                n2755 = local read "AVP 2"() -> (w3642:dbl)
                n2756 = Concatenate Strings("1," ("string"), w3615) -> (w3614:string)
                n2757 = Concatenate Strings("2," ("string"), w3612) -> (w3611:string)
                n2758 = Concatenate Strings("3," ("string"), w3608) -> (w3610:string)
                n2759 = Concatenate Strings("4," ("string"), w3607) -> (w3606:string)
                n2760 = Concatenate Strings("5," ("string"), w3603) -> (w3604:string)
                n2761 = Concatenate Strings("6," ("string"), w3600) -> (w3601:string)
                n2762 = Concatenate Strings("7," ("string"), w3597) -> (w3598:string)
                n2763 = Concatenate Strings("8," ("string"), w3594) -> (w3595:string)
                n2764 = local read "Sample ID"() -> (w3662:string)
                n2765 = case shown="\"xlx\"" "Select File Type" {
                  tunnel: w3620 -> [w3665 w3667 w3669]
                  tunnel: [w3663 w3668 w3670] -> w3619
                  frame "xlx" {
                    n2766 = Concatenate Strings(w3665, ".xls" ("string")) -> (w3663:string)
                  }
                  frame "csv" {
                    n2767 = Concatenate Strings(w3667, ".csv" ("string")) -> (w3668:string)
                  }
                  frame "txt" {
                    n2768 = Concatenate Strings(w3669, ".txt" ("string")) -> (w3670:string)
                  }
                }
                n2769 = local read "Test Date"() -> (w3661:string)
                n2770 = local read "String 45"() -> (w3575:string)
                n2771 = local read "String 31"() -> (w3660:string)
                n2772 = local read "String 32"() -> (w3659:string)
                n2773 = local read "TITTLE"() -> (w3583:string)
                n2774 = Number To Fractional String(number=w3630, width (-)=i16 6, precision (6)=i16 2) -> (F-format string=w3629:string)  [unwired: 1 in]
                n2775 = Number To Fractional String(number=w3644, width (-)=i16 6, precision (6)=i16 2) -> (F-format string=w3650:string)  [unwired: 1 in]
                n2776 = Number To Fractional String(number=w3645, width (-)=i16 6, precision (6)=i16 2) -> (F-format string=w3643:string)  [unwired: 1 in]
                n2777 = Number To Fractional String(number=w3649, width (-)=i16 6, precision (6)=i16 2) -> (F-format string=w3648:string)  [unwired: 1 in]
                n2778 = Number To Fractional String(number=w3641, width (-)=i16 6, precision (6)=i16 2) -> (F-format string=w3639:string)  [unwired: 1 in]
                n2779 = Number To Fractional String(number=w3642, width (-)=i16 6, precision (6)=i16 2) -> (F-format string=w3640:string)  [unwired: 1 in]
                n2780 = Number To Fractional String(number=w3653, width (-)=i16 6, precision (6)=i16 2) -> (F-format string=w3654:string)  [unwired: 1 in]
                n2781 = Number To Fractional String(number=w3657, precision (6)=i16 2) -> (F-format string=w3658:string)  [unwired: 2 in]
                n2782 = local read "s.NO"() -> (w3577:string)
                n2783 = Concatenate Strings("=" ("string"), w3583) -> (w3582:string)
                n2784 = Concatenate Strings("S.No," ("string"), "                                       Parameters" ("string")) -> (w3588:string)
                n2785 = Concatenate Strings(w3655, w3614, w3629, w3655, w3611, w3650, w3655, w3610, w3643, w3655, w3606, w3648, w3655, w3604, w3639, w3655, w3601, w3640, w3655, w3598, w3654, w3655, w3595, w3658) -> (w3617:string)
                n2786 = Concatenate Strings(w3587, "," ("string"), w3575, w3577, w3576, w3659, w3662, w3576, w3660, w3661, w3587) -> (w3585:string)
                n2787 = local read "Tested by"() -> (w3591:string)
                n2788 = local read "String 33"() -> (w3592:string)
                n2789 = Concatenate Strings("," ("string"), "                                                                             " ("string")) -> (w3580:string)
                n2790 = Concatenate Strings(w3582, w3578, w3585, w3578, w3588, w3617, w3578, w3580, w3592, w3591) -> (→"export":string)
                n2791 = String To Path(string=w3619) -> (path=w3626:path)
                n2792 = local read "export"() -> (w3621:string)
                n2793 = call <vilib>:"Write Characters To File.vi"("append to file? (new file:F)"=FALSE, "character string"=w3621, "file path (dialog if empty)"=w3626) -> ()  [unwired: 2 in, 1 out]
              }
            }
          }
          frame Enabled {
          }
        }
        n2794 = case shown="True" "OK Button 17" {
          frame False {
          }
          frame True {
            (unwired) 0  # existing file
            w3879 = "Choose a datalog file to open"  # prompt
            n2795 = local write "OK Button 17"(FALSE ("OK Button 17")) -> ()
            n2796 = local read "String"() -> (w3874:string)
            n2797 = String To Path(string=w3874) -> (path=w3875:path)
            n2798 = File Dialog(6:"*.duf" ("pattern"), 7:w3879, 11:w3875) -> (0:w3866:errorcluster, 3:w3885:path)  [unwired: 4 in, 2 out]
            n2799 = Unbundle(w3866) -> ()  [unwired: 3 out]
            n2800 = Open/Create/Replace File "Open File"(file path (use dialog)=w3885) -> (refnum out=w3877:refnum<file>)  [unwired: 5 in, 2 out]
            n2801 = Strip Path(path=w3885) -> (name=w3883:string)  [unwired: 1 out]
            n2802 = Path To String(path=w3885) -> (string=w3868:string)
            n2803 = while {
              tunnel: w3877 -> [w3889]
              i -> [w3886]
              stop <- w3887 continue-if-true
              (unwired) TRUE ("line mode (F)")
              n2804 = Read from Text File "Read File"(file (use dialog)=w3889) -> (text=w3888:string)  [unwired: 3 in, 3 out]
              n2805 = local write "Numeric 16"(w3886) -> ()
              n2806 = String Length(string=w3888) -> (length=w3891:i32)
              n2807 = Greater?(x=w3891, y=1) -> (0:w3887:bool)
            }
            n2808 = local write "String 29"(w3868) -> ()
            n2809 = Search and Replace String(input string=w3868, search string=".duf", replace string=".dgf" ("replace string (\"\")")) -> (result string=→"String Indicator 4":string)  [unwired: 5 in, 3 out]
            n2810 = Match Pattern(string=w3883, regular expression=".dwm") -> (before substring=w3867:string)  [unwired: 1 in, 3 out]
            "String Indicator" <- w3867
            n2811 = Match Pattern(string=w3868, regular expression=".dwm" ("substring (\"\")")) -> (before substring=w3869:string)  [unwired: 1 in, 3 out]
            "String Indicator 3" <- w3869
            n2812 = local write "TITTLE 2"(w3867) -> ()
            n2813 = String To Path(string=w3869) -> (path=w3876:path)
            "path" <- w3876
            n2814 = call <vilib>:"Read Characters From File.vi"("file path (dialog if empty)"=w3876, "start of read offset (chars.:0)"=60 ("start of read offset (chars.: 0)")) -> ("character string"=→"String Indicator 2":string)  [unwired: 4 in, 3 out]
          }
        }
        n2815 = call <vilib>:"Query Available Printers.vi"() -> ("system configured printers"=w3568:string[])  [unwired: 9 in, 2 out]
        "System Configured Printers 2" <- w3568
        n2816 = local read "OK Button 16"() -> (w3565:bool)
        n2817 = case shown="True" "OK Button 16" {
          frame False {
          }
          frame True {
            n2818 = stacked-sequence {
              frame #0 {
                n2819 = local read "Numeric 16"() -> (w3893:i32)
                n2820 = local write "Numeric 10"(w3893) -> ()
              }
              frame #1 {
                n2821 = local read "String 29"() -> (w3896:string)
                n2822 = String To Path(string=w3896) -> (path=w3895:path)
                n2823 = Open/Create/Replace File "Open File"(file path (use dialog)=w3895) -> (refnum out=w3897:refnum<file>)  [unwired: 5 in, 2 out]
                n2824 = for {
                  N: 16 -> [_]
                  tunnel: w3897 -> [w3904]
                  i -> [w3900]
                  (unwired) TRUE ("line mode (F)")
                  n2825 = Read from Text File "Read File"(file (use dialog)=w3904) -> (text=w3898:string)  [unwired: 3 in, 3 out]
                  n2826 = Match Pattern(string=w3898, regular expression="(") -> (after substring=w3903:string)  [unwired: 1 in, 3 out]
                  n2827 = Match Pattern(string=w3903, regular expression=")") -> (before substring=w3899:string)  [unwired: 1 in, 3 out]
                  n2828 = case shown="1" w3900 {
                    tunnel: w3899 -> [w3905 w3906 _ _ w3907 w3908 w3909 w3911 w3913 w3915 w3917 w3919 w3921 w3923 _]
                    tunnel: w3898 -> [_ _ _ _ _ _ _ _ _ _ _ _ _ _ _]
                    frame 0 {
                      "TITTLE" <- w3905
                    }
                    frame 1 {
                      "Sample ID" <- w3906
                    }
                    frame 2 {
                    }
                    frame 3 {
                    }
                    frame 4 {
                      "Test Date" <- w3907
                    }
                    frame 5 {
                      "Tested by" <- w3908
                    }
                    frame 6 {
                      n2829 = Fract/Exp String To Number(string=w3909) -> (number=→"Humidity before test 2":dbl)  [unwired: 3 in, 1 out]
                    }
                    frame 7 {
                      n2830 = Fract/Exp String To Number(string=w3911) -> (number=→"Temperature before test 2":dbl)  [unwired: 3 in, 1 out]
                    }
                    frame 8 {
                      n2831 = Fract/Exp String To Number(string=w3913) -> (number=→"Humidity after test 2":dbl)  [unwired: 3 in, 1 out]
                    }
                    frame 9 {
                      n2832 = Fract/Exp String To Number(string=w3915) -> (number=→"Temperature after test 2":dbl)  [unwired: 3 in, 1 out]
                    }
                    frame 10 {
                      n2833 = Fract/Exp String To Number(string=w3917) -> (number=→"MWSD 2":dbl)  [unwired: 3 in, 1 out]
                    }
                    frame 11 {
                      n2834 = Fract/Exp String To Number(string=w3919) -> (number=→"AVP 2":dbl)  [unwired: 3 in, 1 out]
                    }
                    frame 12 {
                      n2835 = Fract/Exp String To Number(string=w3921) -> (number=→"HCF 2":dbl)  [unwired: 3 in, 1 out]
                    }
                    frame 13 {
                      n2836 = Fract/Exp String To Number(string=w3923) -> (number=→"WS1.4 2":dbl)  [unwired: 3 in, 1 out]
                    }
                    frame 14, Default {
                    }
                  }
                }
              }
              frame #2 {
              }
            }
            n2837 = local write "OK Button 16"(FALSE ("OK Button 13")) -> ()
          }
        }
        n2838 = Index Array(array=w3568, index="Select Printer 3") -> (element=w3570:string)
        "Selected Printer" <- w3570
        n2839 = case shown="True" w3565 {
          frame False {
          }
          frame True {
            n2840 = flat-sequence {
              frame #0 {
              }
              frame #1 {
                n2841 = Wait (ms)(milliseconds to wait=u32 100) -> ()  [unwired: 1 out]
              }
              frame #2 {
                n2842 = local write "OK Button 16"(FALSE ("Print 3")) -> ()
              }
            }
          }
        }
        n2843 = case shown="True" "Print" {
          tunnel: w3570 -> [_ w3862]
          frame False {
          }
          frame True {
            (unwired) i16 6 ("width (-)")
            (unwired) "TESTED BY : "
            (unwired) "TESTED DATE :"
            (unwired) "SAMPLE ID : "
            (unwired) "SAMPLE DESIGN : "
            w3820 = "\r"
            w3837 = "\r"
            # "add image"
            n2844 = local read "Sample ID"() -> (w3810:string)
            n2845 = local read "Tested by"() -> (w3813:string)
            n2846 = local read "String 34"() -> (w3800:string)
            n2847 = local read "String 45"() -> (w3780:string)
            n2848 = local read "String 35"() -> (w3795:string)
            n2849 = local read "String 37"() -> (w3793:string)
            n2850 = local read "String 32"() -> (w3815:string)
            n2851 = local read "String 36"() -> (w3790:string)
            n2852 = local read "String 31"() -> (w3814:string)
            n2853 = local read "Test Date"() -> (w3811:string)
            n2854 = local read "String 33"() -> (w3816:string)
            n2855 = local read "String 38"() -> (w3786:string)
            n2856 = local read "String 39"() -> (w3783:string)
            n2857 = local write "Print"(FALSE ("Print FF")) -> ()
            n2858 = local read "S 39"() -> (w3798:string)
            n2859 = local read "S 38"() -> (w3805:string)
            n2860 = local read "Temperature before test 2"() -> (w3836:dbl)
            n2861 = local read "Temperature after test 2"() -> (w3826:dbl)
            n2862 = local read "Humidity before test 2"() -> (w3851:dbl)
            n2863 = local read "Humidity after test 2"() -> (w3835:dbl)
            n2864 = local read "MWSD 2"() -> (w3840:dbl)
            n2865 = local read "WS1.4 2"() -> (w3818:dbl)
            n2866 = Concatenate Strings("2)" ("string"), w3800) -> (w3801:string)
            n2867 = Concatenate Strings("3)" ("string"), w3798) -> (w3799:string)
            n2868 = Concatenate Strings("1)" ("string"), w3805) -> (w3804:string)
            n2869 = Concatenate Strings("4)" ("string"), w3795) -> (w3796:string)
            n2870 = Concatenate Strings("5)" ("string"), w3793) -> (w3792:string)
            n2871 = Concatenate Strings("6)" ("string"), w3790) -> (w3789:string)
            n2872 = Concatenate Strings("7)" ("string"), w3786) -> (w3787:string)
            n2873 = Concatenate Strings("8)" ("string"), w3783) -> (w3784:string)
            n2874 = local read "HCF 2"() -> (w3822:dbl)
            n2875 = local read "AVP 2"() -> (w3839:dbl)
            n2876 = local read "s.NO"() -> (w3781:string)
            n2877 = call <vilib>:"New Report.vi"("report type"=enum16{"Standard Report", "HTML"}."Standard Report") -> ("report out"=w3860:refnum<class "NI_report.lvclass">, "error out"=w3859:errorcluster)  [unwired: 13 in]
            n2878 = local read "TITTLE"() -> (w3812:string)
            n2879 = Concatenate Strings(w3837, w3780, w3781, w3837, w3815, w3810, w3837, w3814, w3811, w3837, w3816, w3813, w3837) -> (w3830:string)
            "test by" <- w3830
            n2880 = Number To Fractional String(number=w3836, width (-)=i16 6, precision (6)=i16 2) -> (F-format string=w3825:string)  [unwired: 1 in]
            n2881 = Number To Fractional String(number=w3835, width (-)=i16 6, precision (6)=i16 2) -> (F-format string=w3838:string)  [unwired: 1 in]
            n2882 = Number To Fractional String(number=w3851, width (-)=i16 6, precision (6)=i16 2) -> (F-format string=w3856:string)  [unwired: 1 in]
            n2883 = Number To Fractional String(number=w3840, width (-)=i16 6, precision (6)=i16 2) -> (F-format string=w3842:string)  [unwired: 1 in]
            n2884 = Number To Fractional String(number=w3826, width (-)=i16 6, precision (6)=i16 2) -> (F-format string=w3827:string)  [unwired: 1 in]
            n2885 = Number To Fractional String(number=w3839, width (-)=i16 6, precision (6)=i16 2) -> (F-format string=w3841:string)  [unwired: 1 in]
            n2886 = Number To Fractional String(number=w3822, width (-)=i16 6, precision (6)=i16 2) -> (F-format string=w3821:string)  [unwired: 1 in]
            n2887 = Number To Fractional String(number=w3818, precision (6)=i16 2) -> (F-format string=w3817:string)  [unwired: 2 in]
            n2888 = call-dynamic "Set Report Header Text.vi"("report in"=w3860, "center header text"=w3812, "error in (no error)"=w3859) -> ("report out"=w3831:refnum<class "NI_report.lvclass">, "error out"=w3832:errorcluster)  [unwired: 11 in]
            n2889 = Concatenate Strings(w3820, w3804, w3856, w3820, w3801, w3825, w3820, w3799, w3838, w3820, w3796, w3827, w3820, w3792, w3842, w3820, w3789, w3841, w3820, w3787, w3821, w3820, w3784, w3817) -> (w3808:string)
            "export 2" <- w3808
            n2890 = call-poly <vilib>:"Append Report Text.vi"("report in"=w3831, "text"=w3830, "error in (no error)"=w3832) -> ("report out"=w3834:refnum<class "NI_report.lvclass">, "error out"=w3833:errorcluster)  [unwired: 9 in, 2 out]
            n2891 = local read "test by"() -> (w3807:string)
            n2892 = local read "TITTLE"() -> (w3809:string)
